vi "Create a free text label.vi"   [LabVIEW 2012, in "Scripting Tools.lvlib"]
doc: "Creates a free text label on either the Front Panel or Block Diagram specified in the reference and returns a reference to the new label. The Label defaults to a transparent background."
uses:
  Scripting Tools.lvlib
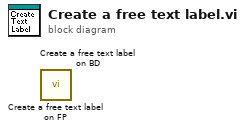
[diagram p0: block diagram]
diagram:
  n1 = call "Create a free text label on FP.vi"() -> ()  [unwired: 10 in, 2 out]
  n2 = call "Create a free text label on BD.vi"() -> ()  [unwired: 10 in, 2 out]
